vi "obtain_background.vi"(8 "error in (no error)":errorcluster, 11 "DL090623TwoDAnalyser in":refnum<class "AnalyserDL090623TwoD.lvclass">) -> (0 "error out":errorcluster, 3 "DL090623TwoDAnalyser out":refnum<class "AnalyserDL090623TwoD.lvclass">)   [LabVIEW 2010, in "AnalyserDL090623TwoD.lvclass"]
uses:
  AnalyserDL090623TwoD.lvclass
  AnalyserDL090623TwoD.lvclass/AnalyserDL090623TwoD.ctl
  common/classes/Image/Image/Image.lvclass
  common/classes/ErrorController/ErrorController/class_data.vi
  common/classes/ErrorController/ErrorController/ErrorController.lvclass
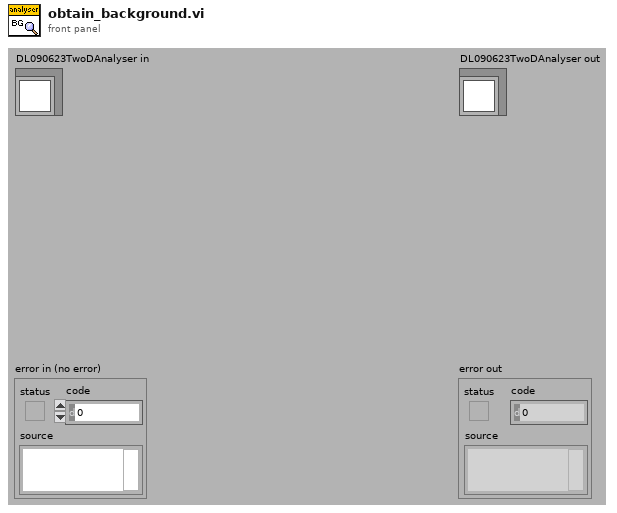
[diagram p1: front panel]
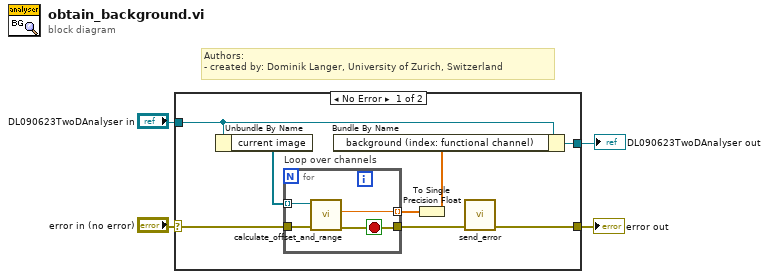
[diagram p0: block diagram]
diagram:
  # "Authors: \n- created by: Dominik Langer, University of Zurich, Switzerland"
  n1 = case shown="No Error" "error in (no error)" {
    selector: "error in (no error)" -> [w7 w18]
    tunnel: [w8 w18] -> w3
    tunnel: [w12 w17] -> w1
    tunnel: "DL090623TwoDAnalyser in" -> [w6 w17]
    frame No Error {
      n2 = Unbundle By Name(w6) -> ("current image"=w5:refnum<class "Image.lvclass">[])
      n3 = for "Loop over channels" {
        tunnel: w5 -> [w15] mode=indexing
        tunnel: [w14] -> w11 mode=indexing
        tunnel: w7 -> [w16]
        tunnel: [w13] -> w9
        stop <- w13 stop-if-true
        n4 = call-dynamic "calculate_offset_and_range.vi"("error in (no error)"=w16, "Image in"=w15) -> ("error out"=w13:errorcluster, "offset / minimum"=w14:dbl)  [unwired: 8 out]
      }
      n5 = To Single Precision Float(number=w11) -> (single precision float=w10:sgl[])
      n6 = Bundle By Name(cluster=w6, "background (index: functional channel)"=w10) -> (w12:refnum<class "AnalyserDL090623TwoD.lvclass">)
      n7 = call "send_error.vi"("error in (no error)"=w9) -> ("error out"=w8:errorcluster)  [unwired: 10 in]
    }
    frame Error {
    }
  }
  "error out" <- w3
  "DL090623TwoDAnalyser out" <- w1
